vi "Timer Page Event Generator.vi"(8 "error in":errorcluster) -> (0 "error out":errorcluster, 3 "Timer Events":T1)   [LabVIEW 2024, in "View.lvlib"]
uses:
  View.lvlib
  Type Defs/Start Event Args--cluster.ctl
  Type Defs/Pause Event Args--cluster.ctl
  Type Defs/Stop Event Args--cluster.ctl
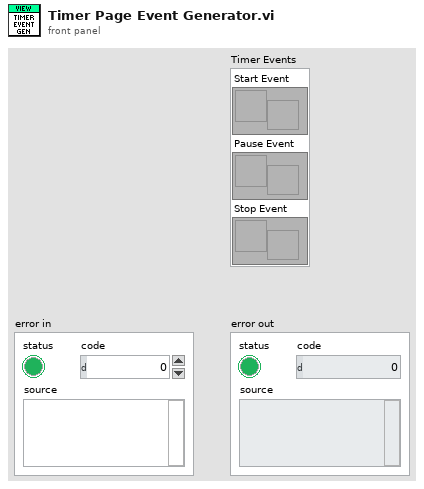
[diagram p1: front panel]
types:
  T1 = cluster{"Start Event":refnum<user-event>, "Pause Event":refnum<user-event>, "Stop Event":refnum<user-event>}
  T2 = typedef "View.lvlib/Stop Event Args--cluster.ctl" = cluster{"None":bool}
  T3 = typedef "View.lvlib/Pause Event Args--cluster.ctl" = cluster{"None":bool}
  T4 = typedef "View.lvlib/Start Event Args--cluster.ctl" = cluster{"None":bool}
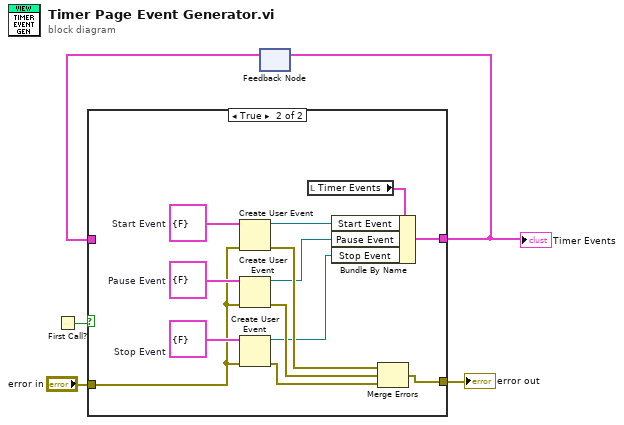
[diagram p0: block diagram]
diagram:
  n1 = First Call?() -> (First Call?: T/F=w5:bool)
  n2 = feedback #1() -> (w4:T1)  [unwired: 1 in]
  n3 = case shown="True" w5 {
    tunnel: [w7 w15] -> w3
    tunnel: w4 -> [w7 _]
    tunnel: "error in" -> [w6 w14]
    tunnel: [w6 w13] -> w1
    frame False {
    }
    frame True {
      w17 = T2 {"None"=FALSE}  # Stop Event
      w18 = T3 {"None"=FALSE}  # Pause Event
      w20 = T4 {"None"=FALSE}  # Start Event
      n4 = Create User Event(user event datatype=w20, error in=w14) -> (user event=w19:refnum<user-event>, error out=w10:errorcluster)
      n5 = Create User Event(user event datatype=w18, error in=w14) -> (user event=w9:refnum<user-event>, error out=w11:errorcluster)
      n6 = Create User Event(user event datatype=w17, error in=w14) -> (user event=w8:refnum<user-event>, error out=w12:errorcluster)
      n7 = local read "Timer Events"() -> (w16:T1)
      n8 = Bundle By Name(cluster=w16, "Start Event"=w19, "Pause Event"=w9, "Stop Event"=w8) -> (w15:T1)
      n9 = Merge Errors(w10, w11, w12) -> (w13:errorcluster)
    }
  }
  "Timer Events" <- w3
  "error out" <- w1
  n10 = feedback-in #1(w3) -> ()
